vi "Measurement UI.vi"() -> ()   [LabVIEW 2021, in "Sweep_Channel Ganging_UI.lvlib"]
uses:
  Sweep_Channel Ganging_UI.lvlib
panel:
  in  "MeasGraphs":enum32{"I-V Sweep", "Hidden Controls"}(tab)
  out "LoadGraph":T1(graph)
  out "SourceGraph":T2(graph)
  in  "Mode of operation":T3(ring)=enum."Perform measurement"
  out "Source sweep values":dbl[](array[numeric])
  in  "Load measure trigger":string
  in  "Load source trigger":string
  out "Source currents":dbl[](array[numeric])
  out "Source voltages":dbl[](array[numeric])
  out "Load currents":dbl[](array[numeric])
  out "Load voltages":dbl[](array[numeric])
  in  "Load resource names":string[](array[string])
  in  "Source resource names":string[](array[string])
  out "Load sweep points":i32
  out "Source sweep points":i32
  in  "ModeOfConfiguration":T4(tab)
  in  "DEVICE POWER":bool=TRUE
  out "Status":string
  in  "Load config power on":string="Load Config"
  in  "POWERON/OFFLOADResourceNames":refnum<k15>[](array[refnum]) caption="RESOURCE NAMES\n(Single/Master & Slave)"
  in  "Source config power on":string="Source Config"
  in  "POWERON/ OFFSOURCEResourceNames":refnum<k15>[](array[refnum]) caption="RESOURCE NAMES\n(Single/Master & Slave)"
  in  "Power on source sense":i32(ring)=1009 caption="SENSE" items=["Local"=1008, "Remote"=1009]
  in  "Power on/off Source voltage/current limit range":dbl=20.0 caption="CURRENT LIMIT" format="%#_6pA"
  in  "Power on/off Source voltage/current level":dbl=6.0 caption="VOLTAGE LEVEL" format="%#_6pV"
  in  "Power on source system configuration":enum32{"Series", "Parallel"}(ring)=enum."Parallel" caption="SYSTEM CONFIG"
  in  "Power on output function":i32(ring)=1006 caption="OUTPUT FUNCTION" items=["DC Voltage"=1006, "DC Current"=1007]
  in  "MeasConfigurations":enum32{"Source Config", "Load Config"}(tab)
  in  "Measurement timeout":dbl=10.0 caption="MEASUREMENT TIMEOUT" format="%.3ps"
  in  "Source voltage/current compensation frequency":dbl(slide)=3530.0 caption="COMP. FREQUENCY" scale=50.0..1000000.0 scale format="%#_6pHz"
  in  "Source voltage/current pole-zero ratio":dbl(slide)=2.0 caption="POLE-ZERO RATIO" scale=0.0625..16.0
  in  "Source voltage/current gain bandwidth":dbl(slide)=2000.0 caption="GAIN BANDWIDTH" scale=10.0..1000000.0 scale format="%#_6pHz"
  in  "Source enable/disable":bool=TRUE caption="Source Enabled/Disabled"
  in  "Source source delay":dbl=0.005 caption="SOURCE DELAY" format="%.3ps"
  in  "PPSResourceNames":refnum<k15>[](array[refnum]) caption="RESOURCE NAMES\n(Single/Master & Slave)"
  in  "Source stop level":dbl=20.0 caption="STOP LEVEL" format="%#_6pV"
  in  "Source transient response":i32(ring)=1038 caption="TRANSIENT RESPONSE" items=["Slow"=1041, "Normal"=1038, "Fast"=1039, "Custom"=1042]
  in  "Power ON/Source sense":i32(ring)=1009 caption="SENSE" items=["Local"=1008, "Remote"=1009]
  in  "Source voltage/current level range":dbl=20.0 caption="VOLTAGE LEVEL RANGE" format="%#_6pV"
  in  "Power ON V/I Source start level":dbl=6.0 caption="START LEVEL" format="%#_6pV"
  in  "Source current/voltage limit high":dbl=25.0 caption="CURRENT LIMIT/LIMIT HIGH" format="%#_6pA"
  in  "Power ON/Source current/voltage limit range":dbl=25.0 caption="CURRENT LIMIT" format="%#_6pA"
  in  "Source limit symmetry":enum32{"Symmetric", "Asymmetric"}(ring)=enum."Asymmetric" caption="LIMIT SYMMETRY"
  in  "Source current/voltage limit low":dbl=-0.6 caption="CURRENT LIMIT LOW" format="%#_6pA"
  in  "Power ON/Source system configuration":enum32{"Series", "Parallel"}(ring)=enum."Parallel" caption="SYSTEM CONFIG"
  in  "Source compliance":string="Compliance"
  in  "Source sourceadapt":string="SourceAdapt"
  in  "Source sweep points/points per decade":i32=4 caption="PTS/PTS PER DECADE"
  in  "Power ON/Source output function":i32(ring)=1006 caption="OUTPUT FUNCTION" items=["DC Voltage"=1006, "DC Current"=1007]
  in  "Source timing":string="Timings"
  in  "Source aperture time":dbl=0.01666 caption="APERTURE TIME" format="%.3ps"
  in  "Source sweep scale":string(combo)="Linear" caption="SCALE"
  in  "Load Voltage/current compensation frequency":dbl(slide)=250000.0 caption="COMP. FREQUENCY" scale=50.0..1000000.0 scale format="%#_6pHz"
  in  "Load Voltage/current pole-zero ratio":dbl(slide)=5.0 caption="POLE-ZERO RATIO" scale=0.0625..16.0
  in  "Load Voltage/current gain bandwidth":dbl(slide)=50000.0 caption="GAIN BANDWIDTH" scale=10.0..1000000.0 scale format="%#_6pHz"
  in  "Load device voltage/current rating":dbl=30.0 caption="DEVICE CURRENT RATING" format="%#_6pA"
  in  "Load Source Trigger":tag caption="SOURCE TRIGGER"
  in  "Load aperture time":dbl=0.01666 caption="APERTURE TIME" format="%.3ps"
  in  "Load Measure Trigger":tag caption="MEASURE TRIGGER"
  in  "Load trigger config":string="Trigger"
  in  "Load timing":string="Timings"
  in  "Load output function":i32(ring)=1007 caption="OUTPUT FUNCTION" items=["DC Voltage"=1006, "DC Current"=1007]
  in  "Load sweep points/points per decade":i32=10 caption="PTS/PTS PER DECADE"
  in  "Load stop level":dbl=10.0 caption="STOP LEVEL" format="%#_6pA"
  in  "Load sourceadapt":string="SourceAdapt"
  in  "Load compliance":string="Compliance"
  in  "Load system configuration":enum32{"Series", "Parallel"}(ring)=enum."Parallel" caption="SYSTEM CONFIG"
  in  "Load current/voltage limit low":dbl caption="VOLTAGE  LIMIT LOW" format="%#_6pV"
  in  "Load limit symmetry":enum32{"Symmetric", "Asymmetric"}(ring) caption="LIMIT SYMMETRY"
  in  "Load current/voltage limit range":dbl=6.0 caption="VOLTAGE LIMIT RANGE" format="%#_6pV"
  in  "Load current/voltage limit high":dbl=inf caption="VOLTAGE LIMIT/LIMIT HIGH" format="%#_6p"
  in  "Load start level":dbl=2.0 caption="START LEVEL" format="%#_6pA"
  in  "Load voltage/current level range":dbl=80.0 caption="CURRENT LEVEL RANGE" format="%#_6pA"
  in  "Load sense":i32(ring)=1009 caption="SENSE" items=["Local"=1008, "Remote"=1009]
  in  "Load transient response":i32(ring)=1038 caption="TRANSIENT RESPONSE" items=["Slow"=1041, "Normal"=1038, "Fast"=1039, "Custom"=1042]
  in  "LoadResourceNames":refnum<k15>[](array[refnum]) caption="RESOURCE NAMES\n(Single/Master & Slave)"
  in  "Load source delay":dbl=0.005 caption="SOURCE DELAY" format="%.3ps"
  in  "Load sweep scale":string(combo)="Linear" caption="SCALE"
  in  "Load enable/disable":bool=TRUE caption="Load Enabled/Disabled"
  out "Eload status":string
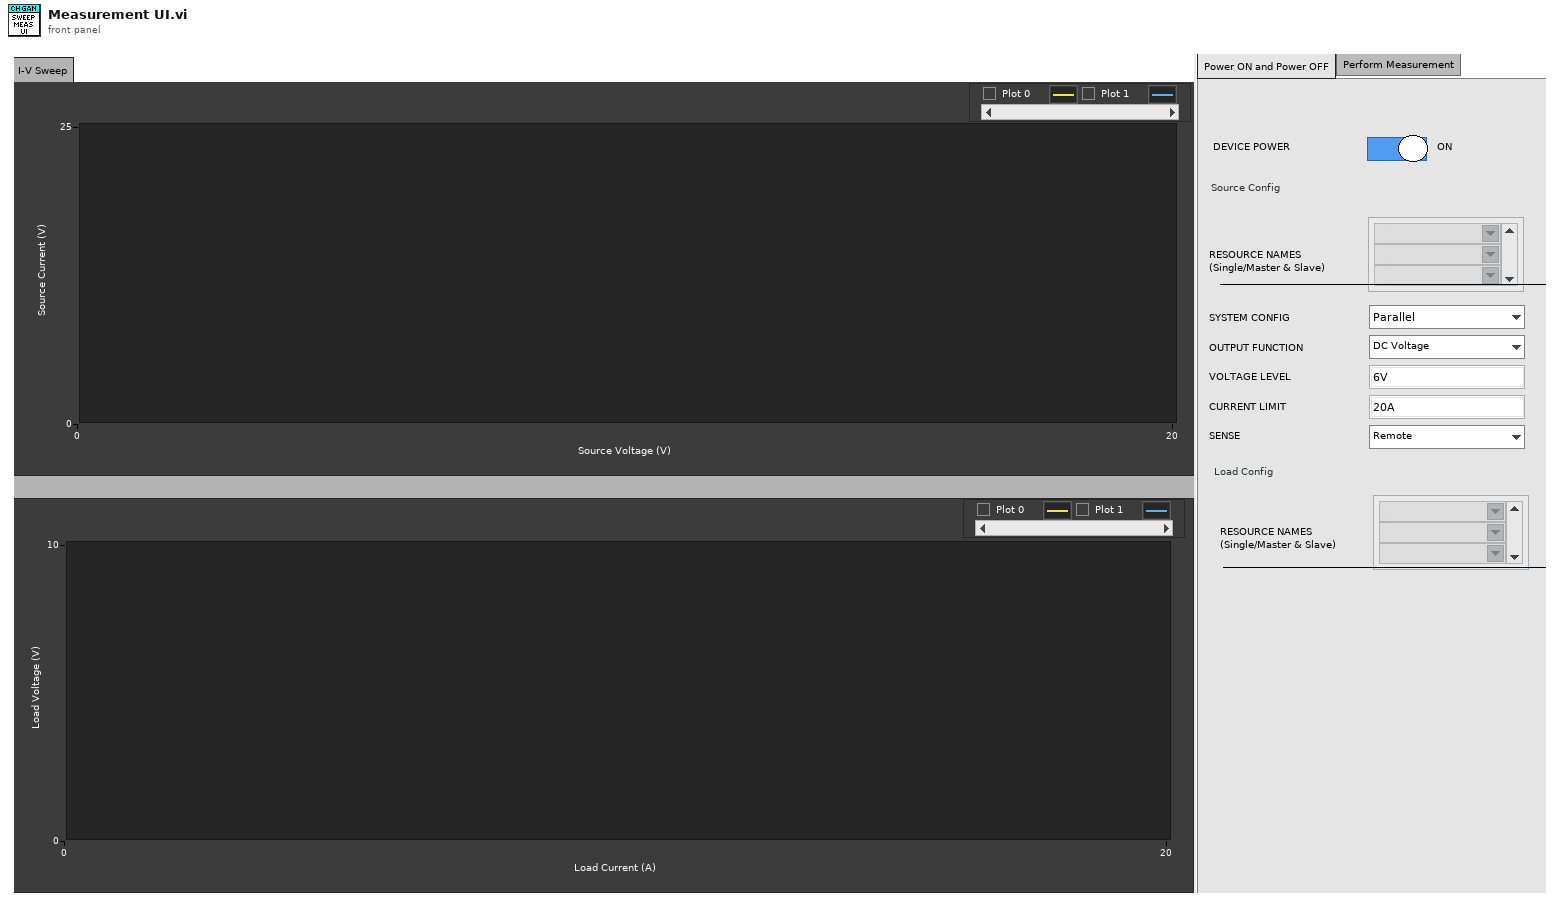
[diagram p1: front panel]
types:
  T1 = cluster{"Ganged load voltages":dbl[], "Ganged load currents":dbl[]}[]
  T2 = cluster{"Ganged source currents":dbl[], "Ganged source voltages":dbl[]}[]
  T3 = enum32{"Power on the DUT", "Perform measurement", "Power off the DUT"}
  T4 = enum32{"Power ON and Power OFF", "Perform Measurement"}
  T5 = enum8{"Enabled", "Disabled", "Disabled and Grayed Out"}
  T6 = cluster{"Source currents":dbl[], "Source voltages":dbl[]}
  T7 = cluster{"Load voltages":dbl[], "Load currents":dbl[]}
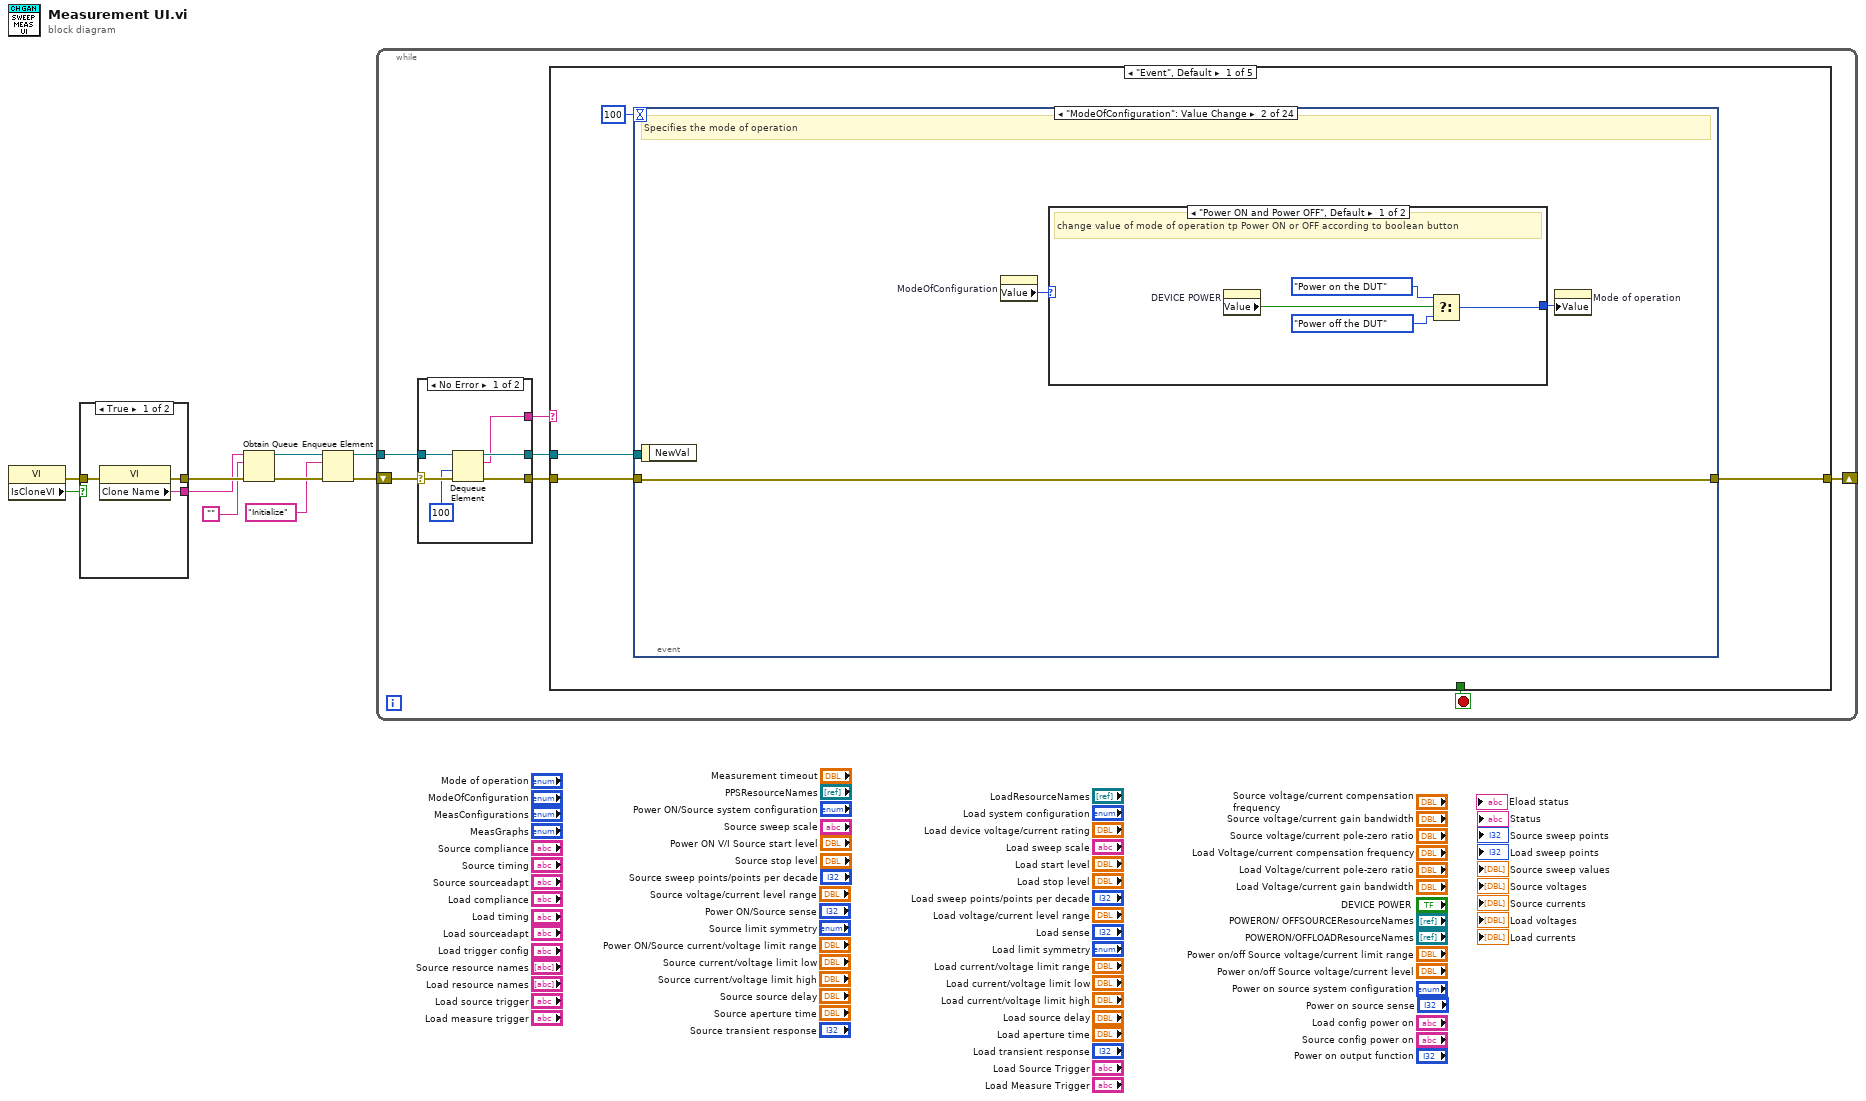
[diagram p0: block diagram]
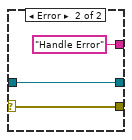
[diagram p2: hidden frame]
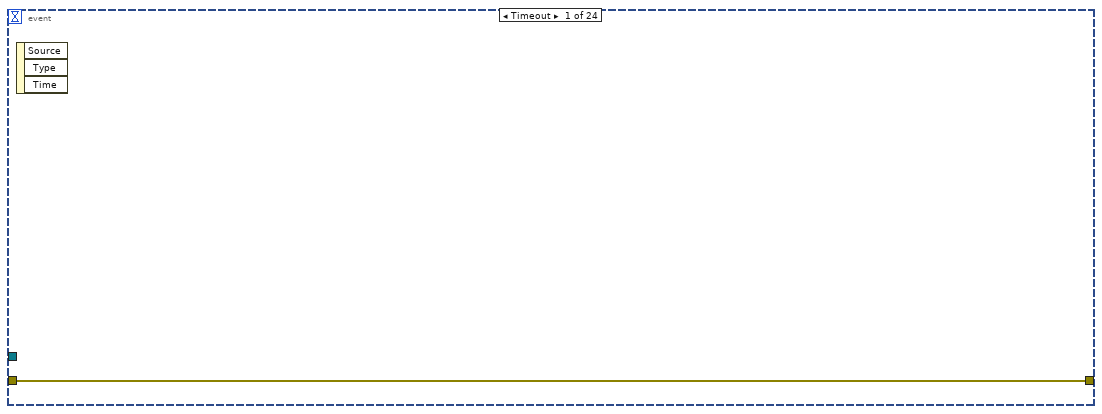
[diagram p3: hidden frame]
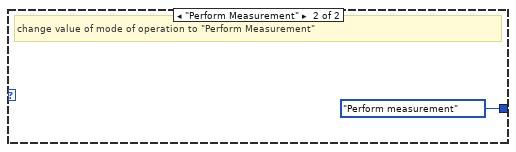
[diagram p4: hidden frame]
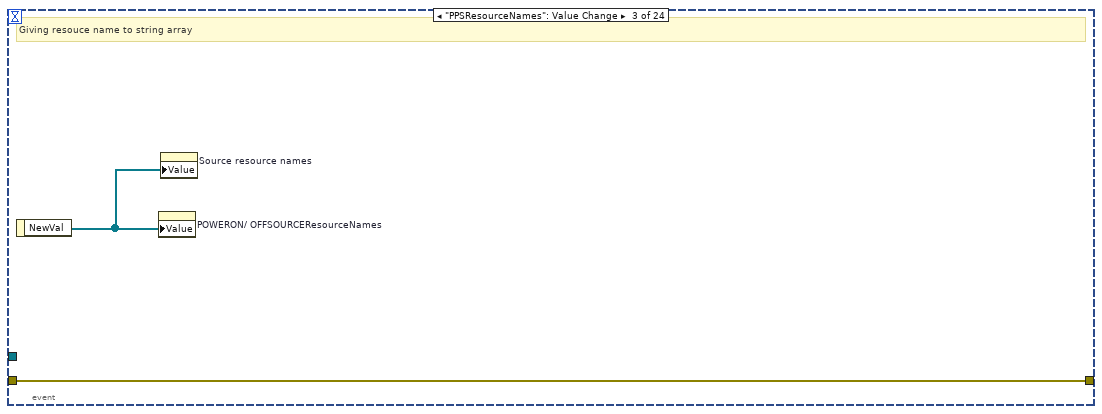
[diagram p5: hidden frame]
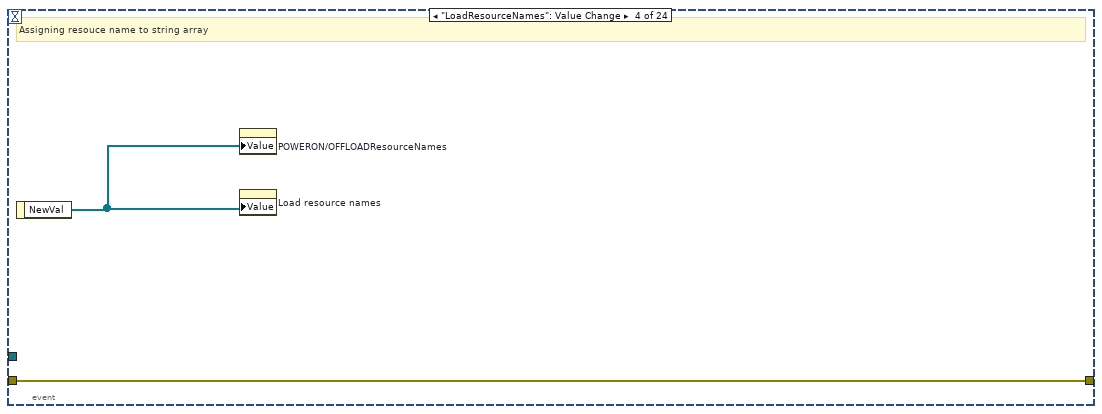
[diagram p6: hidden frame]
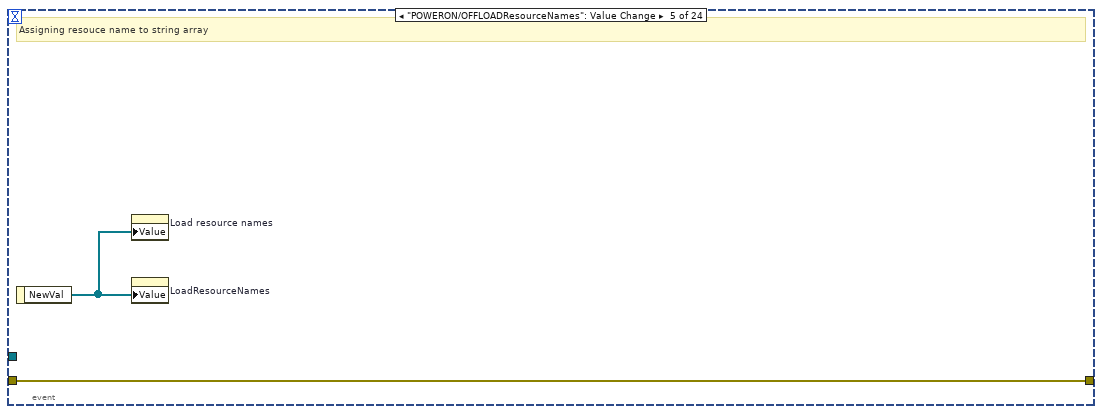
[diagram p7: hidden frame]
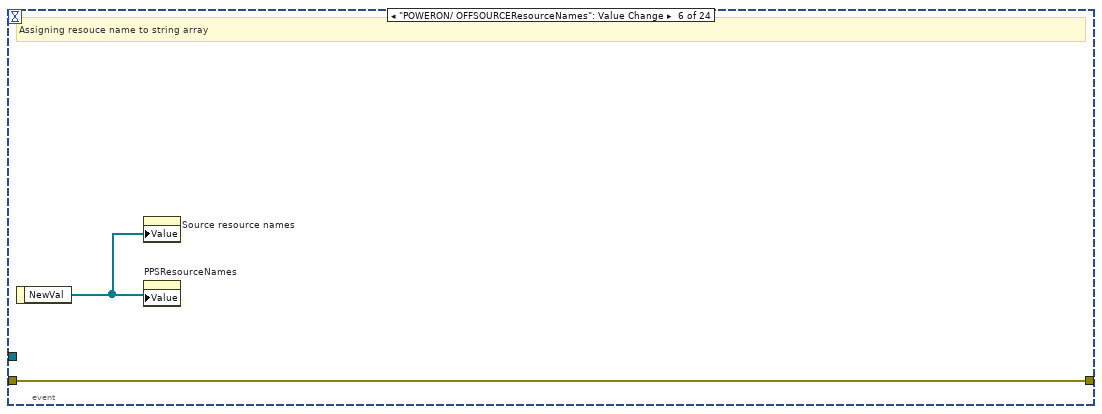
[diagram p8: hidden frame]
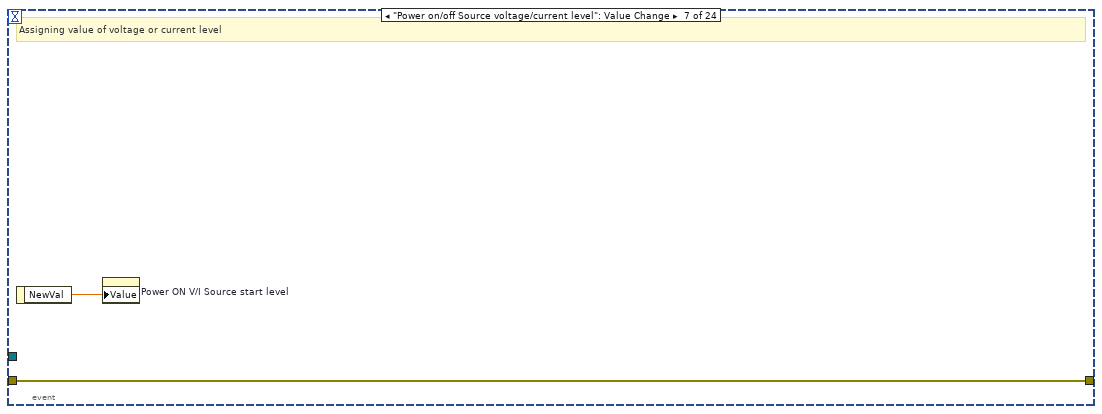
[diagram p9: hidden frame]
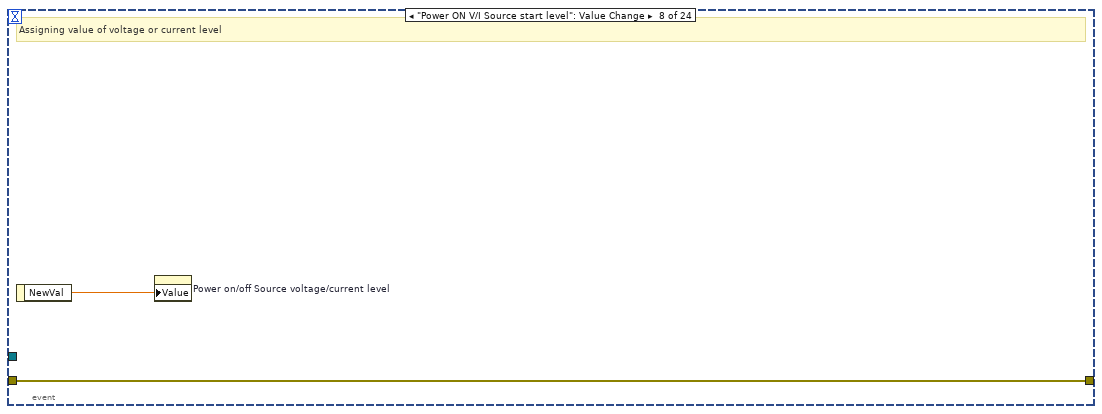
[diagram p10: hidden frame]
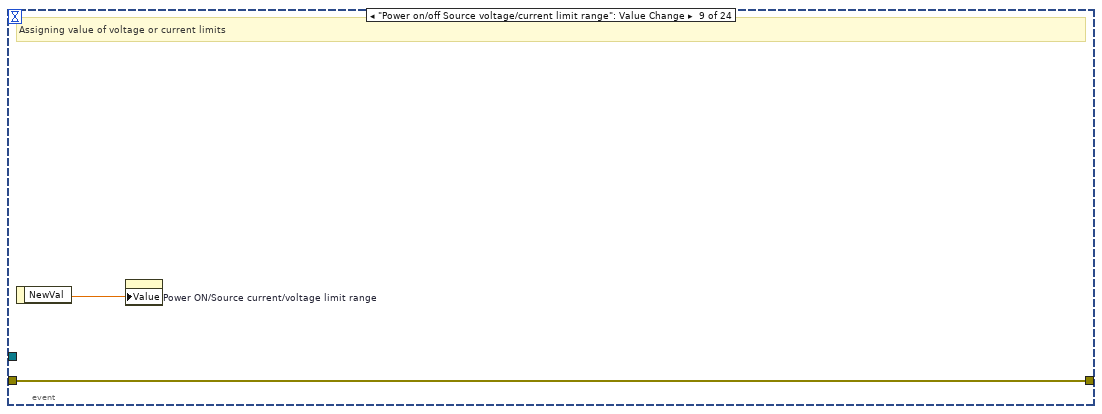
[diagram p11: hidden frame]
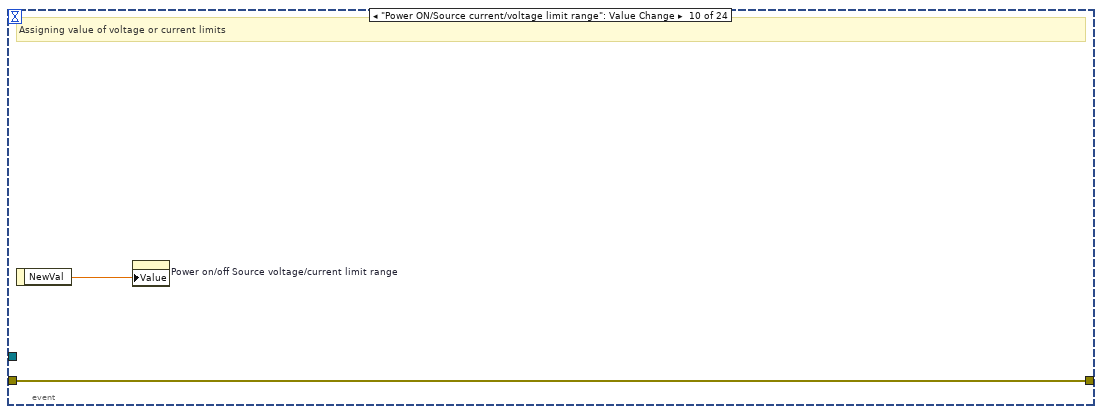
[diagram p12: hidden frame]
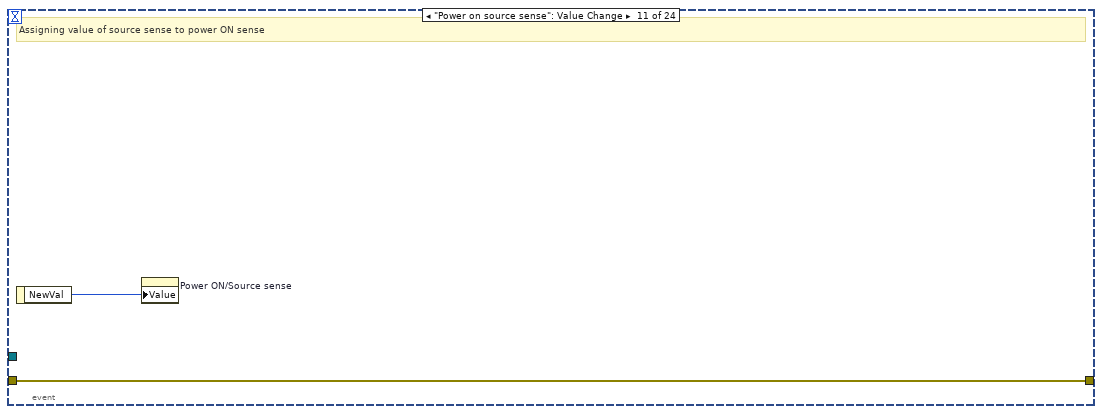
[diagram p13: hidden frame]
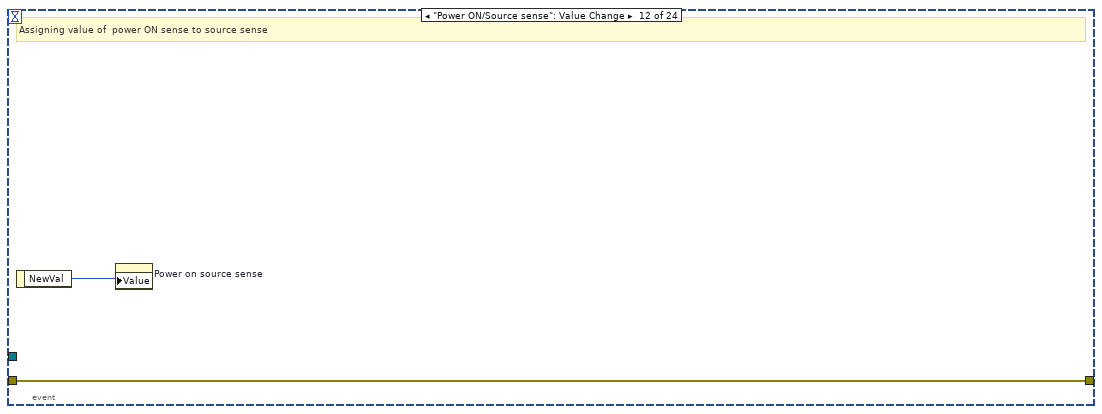
[diagram p14: hidden frame]
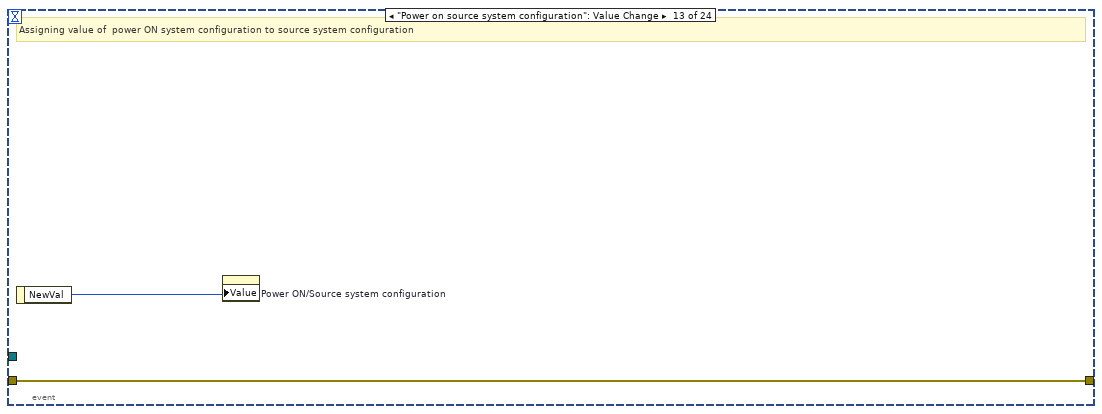
[diagram p15: hidden frame]
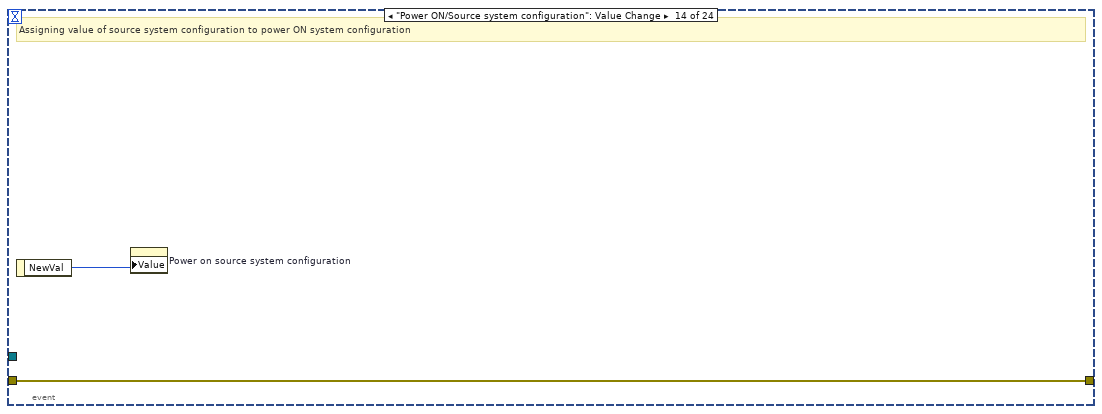
[diagram p16: hidden frame]
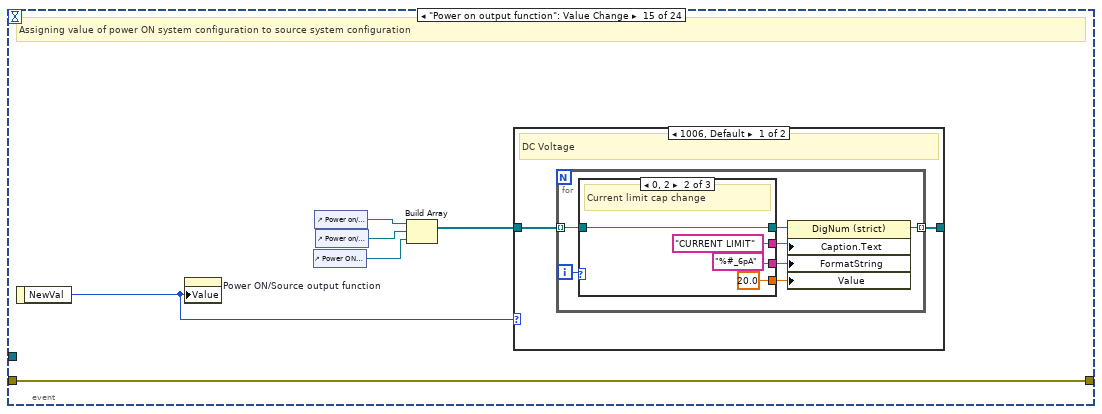
[diagram p17: hidden frame]
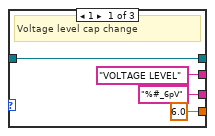
[diagram p18: hidden frame]
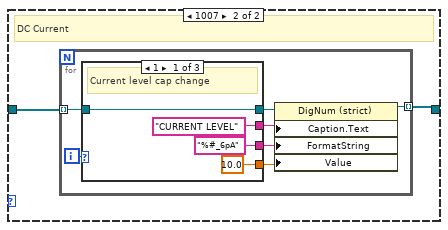
[diagram p20: hidden frame]
diagram:
  n1 = property class="VI"() -> (error out=w1:errorcluster, "IsCloneVI"=w2:bool)  [unwired: 2 in, 1 out]
  n2 = case shown="True" w2 {
    tunnel: [w13 w16] -> w10
    tunnel: [w12 w15] -> w9
    tunnel: w1 -> [w11 w14]
    frame True {
      n3 = property class="VI"(error in=w11) -> (error out=w13:errorcluster, "Clone Name"=w12:string)  [unwired: 1 in, 1 out]
    }
    frame False {
      n4 = property class="VI"(error in=w14) -> (error out=w16:errorcluster, "Name"=w15:string)  [unwired: 1 in, 1 out]
    }
  }
  n5 = Obtain Queue(name (unnamed)=w9, element data type="", error in (no error)=w10) -> (queue out=w6:refnum<queue>, error out=w8:errorcluster)  [unwired: 2 in, 1 out]
  n6 = Enqueue Element(queue=w6, element="Initialize", error in (no error)=w8) -> (queue out=w5:refnum<queue>, error out=w7:errorcluster)  [unwired: 1 in, 1 out]
  n7 = while {
    shift-right: [w18] -> _
    shift-left: w7 -> [w23]
    tunnel: w5 -> [w21]
    stop <- w17 stop-if-true
    n8 = case shown="No Error" w23 {
      selector: w23 -> [w29 w32]
      tunnel: [w28 w32] -> w22
      tunnel: w21 -> [w27 w31]
      tunnel: [w26 w31] -> w20
      tunnel: [w25 "Handle Error"] -> w19
      frame No Error {
        n9 = Dequeue Element(queue=w27, timeout in ms (-1)=100, error in (no error)=w29) -> (queue out=w26:refnum<queue>, element=w25:string, error out=w28:errorcluster)  [unwired: 1 out]
      }
      frame Error {
      }
    }
    n10 = case shown="\"Event\", Default" w19 {
      tunnel: w22 -> [w35 w303 w333 w401 w402]
      tunnel: w20 -> [w33 _ _ w399 _]
      tunnel: [w36 w303 w333 w396 w402] -> w18
      tunnel: [_ _ _ TRUE _] -> w17
      frame "Event", Default {
        n11 = event shown="[1] \"ModeOfConfiguration\": Value Change" {
          selector: _ -> [_ _ _ _ _ _ _ _ _ _ _ _ _ _ _ _ _ _ _ _ _ _ _ _]
          dyn-events: _ -> [_ _ _ _ _ _ _ _ _ _ _ _ _ _ _ _ _ _ _ _ _ _ _ _]
          timeout: 100 -> [_ _ _ _ _ _ _ _ _ _ _ _ _ _ _ _ _ _ _ _ _ _ _ _]
          tunnel: [w37 w38 w47 w49 w51 w53 w55 w57 w58 w61 w62 w64 w66 w68 w75 w111 w188 w274 w276 w278 w283 _ _ w298] -> w36
          tunnel: w35 -> [w37 w38 w47 w49 w51 w53 w55 w57 w58 w61 w62 w64 w66 w68 w75 w112 w189 w274 w276 w278 w283 _ _ w299]
          tunnel: w33 -> [_ _ _ _ _ _ _ _ _ _ _ _ _ _ _ _ _ _ _ _ _ _ _ w297]
          event Timeout {
            n12 = event-data() -> ()  [unwired: 1 in, 3 out]
          }
          event "ModeOfConfiguration": Value Change {
            # "Specifies the mode of operation"
            n13 = event-data() -> ()  [unwired: 1 in, 1 out]
            n14 = property on="ModeOfConfiguration" class="TabCtl (strict)"() -> ("Value"=w40:T4)  [unwired: 2 in, 2 out]
            n15 = case shown="\"Power ON and Power OFF\", Default" w40 {
              tunnel: [w43 T3."Perform measurement" ("Mode of operation")] -> w39
              frame "Power ON and Power OFF", Default {
                # "change value of mode of operation tp Power ON or OFF according to boolean button"
                n16 = property on="DEVICE POWER" class="Bool (strict)"() -> ("Value"=w41:bool)  [unwired: 2 in, 2 out]
                n17 = Select(t=T3."Power on the DUT" ("Mode of operation"), s=w41, f=T3."Power off the DUT" ("Mode of operation")) -> (s? t:f=w43:T3)
              }
              frame "Perform Measurement" {
                # "change value of mode of operation to \"Perform Measurement\""
              }
            }
            n18 = property on="Mode of operation" class="Enum (strict)"("Value"=w39) -> ()  [unwired: 2 in, 2 out]
          }
          event "PPSResourceNames": Value Change {
            # "Giving resouce name to string array"
            n19 = event-data() -> ("NewVal"=w46:refnum<k15>[])  [unwired: 1 in]
            n20 = property on="POWERON/ OFFSOURCEResourceNames" class="Arr (strict)"("Value"=w46) -> ()  [unwired: 2 in, 2 out]
            n21 = property on="Source resource names" class="Arr (strict)"("Value"=w46) -> ()  [unwired: 2 in, 2 out]
          }
          event "LoadResourceNames": Value Change {
            # "Assigning resouce name to string array"
            n22 = event-data() -> ("NewVal"=w48:refnum<k15>[])  [unwired: 1 in]
            n23 = property on="POWERON/OFFLOADResourceNames" class="Arr (strict)"("Value"=w48) -> ()  [unwired: 2 in, 2 out]
            n24 = property on="Load resource names" class="Arr (strict)"("Value"=w48) -> ()  [unwired: 2 in, 2 out]
          }
          event "POWERON/OFFLOADResourceNames": Value Change {
            # "Assigning resouce name to string array"
            n25 = event-data() -> ("NewVal"=w50:refnum<k15>[])  [unwired: 1 in]
            n26 = property on="Load resource names" class="Arr (strict)"("Value"=w50) -> ()  [unwired: 2 in, 2 out]
            n27 = property on="LoadResourceNames" class="Arr (strict)"("Value"=w50) -> ()  [unwired: 2 in, 2 out]
          }
          event "POWERON/ OFFSOURCEResourceNames": Value Change {
            # "Assigning resouce name to string array"
            n28 = event-data() -> ("NewVal"=w52:refnum<k15>[])  [unwired: 1 in]
            n29 = property on="Source resource names" class="Arr (strict)"("Value"=w52) -> ()  [unwired: 2 in, 2 out]
            n30 = property on="PPSResourceNames" class="Arr (strict)"("Value"=w52) -> ()  [unwired: 2 in, 2 out]
          }
          event "Power on/off Source voltage/current level": Value Change {
            # "Assigning value of voltage or current level"
            n31 = event-data() -> ("NewVal"=w54:dbl)  [unwired: 1 in]
            n32 = property on="Power ON V/I Source start level" class="DigNum (strict)"("Value"=w54) -> ()  [unwired: 2 in, 2 out]
          }
          event "Power ON V/I Source start level": Value Change {
            # "Assigning value of voltage or current level"
            n33 = event-data() -> ("NewVal"=w56:dbl)  [unwired: 1 in]
            n34 = property on="Power on/off Source voltage/current level" class="DigNum (strict)"("Value"=w56) -> ()  [unwired: 2 in, 2 out]
          }
          event "Power on/off Source voltage/current limit range": Value Change {
            # "Assigning value of voltage or current limits"
            n35 = event-data() -> ("NewVal"=w59:dbl)  [unwired: 1 in]
            n36 = property on="Power ON/Source current/voltage limit range" class="DigNum (strict)"("Value"=w59) -> ()  [unwired: 2 in, 2 out]
          }
          event "Power ON/Source current/voltage limit range": Value Change {
            # "Assigning value of voltage or current limits"
            n37 = event-data() -> ("NewVal"=w60:dbl)  [unwired: 1 in]
            n38 = property on="Power on/off Source voltage/current limit range" class="DigNum (strict)"("Value"=w60) -> ()  [unwired: 2 in, 2 out]
          }
          event "Power on source sense": Value Change {
            # "Assigning value of source sense to power ON sense"
            n39 = event-data() -> ("NewVal"=w63:i32)  [unwired: 1 in]
            n40 = property on="Power ON/Source sense" class="Ring (strict)"("Value"=w63) -> ()  [unwired: 2 in, 2 out]
          }
          event "Power ON/Source sense": Value Change {
            # "Assigning value of  power ON sense to source sense"
            n41 = event-data() -> ("NewVal"=w65:i32)  [unwired: 1 in]
            n42 = property on="Power on source sense" class="Ring (strict)"("Value"=w65) -> ()  [unwired: 2 in, 2 out]
          }
          event "Power on source system configuration": Value Change {
            # "Assigning value of  power ON system configuration to source system configuration"
            n43 = event-data() -> ("NewVal"=w67:enum32{"Series", "Parallel"})  [unwired: 1 in]
            n44 = property on="Power ON/Source system configuration" class="Enum (strict)"("Value"=w67) -> ()  [unwired: 2 in, 2 out]
          }
          event "Power ON/Source system configuration": Value Change {
            # "Assigning value of source system configuration to power ON system configuration"
            n45 = event-data() -> ("NewVal"=w69:enum32{"Series", "Parallel"})  [unwired: 1 in]
            n46 = property on="Power on source system configuration" class="Enum (strict)"("Value"=w69) -> ()  [unwired: 2 in, 2 out]
          }
          event "Power on output function": Value Change {
            # "Assigning value of power ON system configuration to source system configuration"
            n47 = event-data() -> ("NewVal"=w74:i32)  [unwired: 1 in]
            n48 = property on="Power ON/Source output function" class="Ring (strict)"("Value"=w74) -> ()  [unwired: 2 in, 2 out]
            n49 = control-ref of="Power ON/Source current/voltage limit range"() -> (w70:refnum<vi>)
            n50 = control-ref of="Power on/off Source voltage/current limit range"() -> (w73:refnum<vi>)
            n51 = control-ref of="Power on/off Source voltage/current level"() -> (w72:refnum<vi>)
            n52 = Build Array(w73, w72, w70) -> (w71:refnum<vi>[])
            n53 = case shown="1006, Default" w74 {
              tunnel: w71 -> [w77 w94]
              tunnel: [w76 w93] -> _
              frame 1006, Default {
                # "DC Voltage"
                n54 = for {
                  tunnel: w77 -> [w82] mode=indexing
                  tunnel: [w78] -> w76 mode=indexing
                  i -> [w84]
                  n55 = case shown="0, 2" w84 {
                    tunnel: [w88 w92 _] -> w83
                    tunnel: w82 -> [w88 w92 _]
                    tunnel: ["VOLTAGE LEVEL" ("Caption.Text") "CURRENT LIMIT" ("Caption.Text") _] -> w81
                    tunnel: ["%#_6pV" ("Format String") "%#_6pA" ("Format String") _] -> w80
                    tunnel: [6.0 ("Value") 20.0 ("Value") _] -> w79
                    frame 1 {
                      # "Voltage level cap change"
                    }
                    frame 0, 2 {
                      # "Current limit cap change"
                    }
                    frame Default {
                    }
                  }
                  n56 = property class="DigNum (strict)"(reference=w83, "Caption.Text"=w81, "FormatString"=w80, "Value"=w79) -> (reference out=w78:refnum<vi>)  [unwired: 1 in, 1 out]
                }
              }
              frame 1007 {
                # "DC Current"
                n57 = for {
                  tunnel: w94 -> [w99] mode=indexing
                  tunnel: [w95] -> w93 mode=indexing
                  i -> [w101]
                  n58 = case shown="1" w101 {
                    tunnel: [w105 w109 _] -> w100
                    tunnel: w99 -> [w105 w109 _]
                    tunnel: ["CURRENT LEVEL" ("Caption.Text") "VOLTAGE LIMIT" ("Caption.Text") _] -> w98
                    tunnel: ["%#_6pA" ("Format String") "%#_6pV" ("Format String") _] -> w97
                    tunnel: [10.0 ("Value") 20.0 ("Value") _] -> w96
                    frame 1 {
                      # "Current level cap change"
                    }
                    frame 0, 2 {
                      # "Voltage limit cap change"
                    }
                    frame Default {
                    }
                  }
                  n59 = property class="DigNum (strict)"(reference=w100, "Caption.Text"=w98, "FormatString"=w97, "Value"=w96) -> (reference out=w95:refnum<vi>)  [unwired: 1 in, 1 out]
                }
              }
            }
          }
          event "Power ON/Source output function": Value Change {
            # "Assigning value of source system configuration to power ON system configuration and change in caption of few of the controls"
            n60 = event-data() -> ("NewVal"=w110:i32)  [unwired: 1 in]
            n61 = property on="Power on output function" class="Ring (strict)"("Value"=w110) -> ()  [unwired: 2 in, 2 out]
            n62 = control-ref of="Power ON V/I Source start level"() -> (w120:refnum<vi>)
            n63 = control-ref of="Source stop level"() -> (w119:refnum<vi>)
            n64 = control-ref of="Source voltage/current level range"() -> (w118:refnum<vi>)
            n65 = control-ref of="Power ON/Source current/voltage limit range"() -> (w117:refnum<vi>)
            n66 = control-ref of="Source current/voltage limit low"() -> (w116:refnum<vi>)
            n67 = control-ref of="Source current/voltage limit high"() -> (w115:refnum<vi>)
            n68 = Build Array(w120, w119, w118, w117, w116, w115) -> (w114:refnum<vi>[])
            n69 = case shown="1006, Default" w110 {
              tunnel: w114 -> [w122 w155]
              tunnel: [w121 w154] -> w113
              frame 1006, Default {
                # "DC Voltage"
                n70 = for {
                  tunnel: w122 -> [w127] mode=indexing
                  tunnel: [w123] -> w121 mode=indexing
                  i -> [w129]
                  n71 = case shown="3" w129 {
                    tunnel: [w133 w137 w141 w145 w148 w152 _] -> w128
                    tunnel: w127 -> [w133 w137 w141 w145 w148 w152 _]
                    tunnel: ["START LEVEL" ("Caption.Text") "STOP LEVEL" ("Caption.Text") "VOLTAGE LEVEL RANGE" ("Caption.Text") "CURRENT LIMIT RANGE" ("Caption.Text") "CURRENT LIMIT LOW" ("Caption.Text") "CURRENT LIMIT/LIMIT HIGH" ("Caption.Text") _] -> w126
                    tunnel: ["%#_6pV" ("Format String") "%#_6pV" ("Format String") "%#_6pV" ("Format String") "%#_6pA" ("Format String") "%#_6pA" ("Format String") "%#_6pA" ("Format String") _] -> w125
                    tunnel: [1.0 ("Value") 20.0 ("Value") 20.0 ("Value") 15.0 ("Value") -0.6 ("Value") 15.0 ("Value") _] -> w124
                    frame 0 {
                      # "Start voltage level cap change"
                    }
                    frame 1 {
                      # "Stop voltage level cap change"
                    }
                    frame 2 {
                      # "Voltage level range cap change"
                    }
                    frame 3 {
                      # "Current limit range cap change"
                    }
                    frame 4 {
                      # "Current limit low cap change"
                    }
                    frame 5 {
                      # "Current limit high cap change"
                    }
                    frame Default {
                    }
                  }
                  n72 = property class="DigNum (strict)"(reference=w128, "Caption.Text"=w126, "FormatString"=w125, "Value"=w124) -> (reference out=w123:refnum<vi>)  [unwired: 1 in, 1 out]
                }
              }
              frame 1007 {
                # "DC Current"
                n73 = for {
                  tunnel: w155 -> [w160] mode=indexing
                  tunnel: [w156] -> w154 mode=indexing
                  i -> [w162]
                  n74 = case shown="3" w162 {
                    tunnel: [w166 w170 w174 w178 w181 w185 _] -> w161
                    tunnel: w160 -> [w166 w170 w174 w178 w181 w185 _]
                    tunnel: ["START LEVEL" ("Caption.Text") "STOP LEVEL" ("Caption.Text") "CURRENT LEVEL RANGE" ("Caption.Text") "VOLTAGE LIMIT RANGE" ("Caption.Text") "VOLTAGE  LIMIT LOW" ("Caption.Text") "VOLTAGE LIMIT/LIMIT HIGH" ("Caption.Text") _] -> w159
                    tunnel: ["%#_6pA" ("Format String") "%#_6pA" ("Format String") "%#_6pA" ("Format String") "%#_6pV" ("Format String") "%#_6pV" ("Format String") "%#_6pV" ("Format String") _] -> w158
                    tunnel: [1.0 ("Value") 25.0 ("Value") 25.0 ("Value") 12.0 ("Value") -0.6 ("Value") 12.0 ("Value") _] -> w157
                    frame 0 {
                      # "Current start level cap change"
                    }
                    frame 1 {
                      # "Current stop level cap change"
                    }
                    frame 2 {
                      # "Current level range cap change"
                    }
                    frame 3 {
                      # "Voltage limit range cap change"
                    }
                    frame 4 {
                      # "Voltage limit low cap change"
                    }
                    frame 5 {
                      # "Voltage limit high cap change"
                    }
                    frame Default {
                    }
                  }
                  n75 = property class="DigNum (strict)"(reference=w161, "Caption.Text"=w159, "FormatString"=w158, "Value"=w157) -> (reference out=w156:refnum<vi>)  [unwired: 1 in, 1 out]
                }
              }
            }
            n76 = Close Reference(reference=w113, error in (no error)=w112) -> (error out=w111:errorcluster)
          }
          event "Load output function": Value Change {
            # "Change in caption of few of the controls"
            n77 = event-data() -> ("NewVal"=w198:i32)  [unwired: 1 in]
            n78 = control-ref of="Load device voltage/current rating"() -> (w187:refnum<vi>)
            n79 = control-ref of="Load start level"() -> (w197:refnum<vi>)
            n80 = control-ref of="Load stop level"() -> (w196:refnum<vi>)
            n81 = control-ref of="Load voltage/current level range"() -> (w194:refnum<vi>)
            n82 = control-ref of="Load current/voltage limit range"() -> (w193:refnum<vi>)
            n83 = control-ref of="Load current/voltage limit low"() -> (w192:refnum<vi>)
            n84 = control-ref of="Load current/voltage limit high"() -> (w191:refnum<vi>)
            n85 = Build Array(w197, w196, w194, w193, w192, w191, w187) -> (w195:refnum<vi>[])
            n86 = case shown="1007, Default" w198 {
              tunnel: w195 -> [w200 w237]
              tunnel: [w199 w236] -> w190
              frame 1006 {
                # "DC Voltage"
                n87 = for {
                  tunnel: w200 -> [w205] mode=indexing
                  tunnel: [w201] -> w199 mode=indexing
                  i -> [w207]
                  n88 = case shown="0" w207 {
                    tunnel: [w211 w215 w219 w223 w226 w230 w235 _] -> w206
                    tunnel: w205 -> [w211 w215 w219 w223 w226 w230 w235 _]
                    tunnel: ["START LEVEL" ("Caption.Text") "STOP LEVEL" ("Caption.Text") "VOLTAGE LEVEL RANGE" ("Caption.Text") "CURRENT LIMIT RANGE" ("Caption.Text") "CURRENT LIMIT LOW" ("Caption.Text") "CURRENT LIMIT/LIMIT HIGH" ("Caption.Text") "DEVICE VOLTAGE RATING" ("Caption.Text") _] -> w204
                    tunnel: ["%#_6pV" ("Format String") "%#_6pV" ("Format String") "%#_6pV" ("Format String") "%#_6pA" ("Format String") "%#_6pA" ("Format String") "%#_6pA" ("Format String") "%#_6pV" ("Format String") _] -> w203
                    tunnel: [1.0 ("Value") 60.0 ("Value") 60.0 ("Value") 4.0 ("Value") 0.0 ("Value") 4.0 ("Value") 25.0 ("Value") _] -> w202
                    frame 0 {
                      # "Start voltage level cap change"
                    }
                    frame 1 {
                      # "Stop voltage level cap change"
                    }
                    frame 2 {
                      # "Voltage level range cap change"
                    }
                    frame 3 {
                      # "Current limit range cap change"
                    }
                    frame 4 {
                      # "Current limit low cap change"
                    }
                    frame 5 {
                      # "Current limit high cap change"
                    }
                    frame 6 {
                      # "Device rating cap change"
                    }
                    frame Default {
                    }
                  }
                  n89 = property class="DigNum (strict)"(reference=w206, "Caption.Text"=w204, "FormatString"=w203, "Value"=w202) -> (reference out=w201:refnum<vi>)  [unwired: 1 in, 1 out]
                }
              }
              frame 1007, Default {
                # "DC Current"
                n90 = for {
                  tunnel: w237 -> [w242] mode=indexing
                  tunnel: [w238] -> w236 mode=indexing
                  i -> [w244]
                  n91 = case shown="0" w244 {
                    tunnel: [w248 w252 w256 w260 w263 w268 w271 _] -> w243
                    tunnel: w242 -> [w248 w252 w256 w260 w263 w268 w271 _]
                    tunnel: ["START LEVEL" ("Caption.Text") "STOP LEVEL" ("Caption.Text") "CURRENT LEVEL RANGE" ("Caption.Text") "VOLTAGE LIMIT RANGE" ("Caption.Text") "VOLTAGE  LIMIT LOW" ("Caption.Text") "VOLTAGE LIMIT/LIMIT HIGH" ("Caption.Text") "DEVICE CURRENT RATING" ("Caption.Text") _] -> w241
                    tunnel: ["%#_6pA" ("Format String") "%#_6pA" ("Format String") "%#_6pA" ("Format String") "%#_6pV" ("Format String") "%#_6pV" ("Format String") "%#_6p" ("Format String") "%#_6pA" ("Format String") _] -> w240
                    tunnel: [1.0 ("Value") 40.0 ("Value") 40.0 ("Value") 6.0 ("Value") 0.0 ("Value") w266 30.0 ("Value") _] -> w239
                    frame 0 {
                      # "Start current level cap change"
                    }
                    frame 1 {
                      # "Stop current level cap change"
                    }
                    frame 2 {
                      # "Current level range cap change"
                    }
                    frame 3 {
                      # "Voltage limit range cap change"
                    }
                    frame 4 {
                      # "Voltage limit low cap change"
                    }
                    frame 5 {
                      # "Voltage limit high cap change"
                      n92 = Reciprocal(x=0.0) -> (1/x=w266:dbl)
                    }
                    frame 6 {
                      # "Device rating cap change"
                    }
                    frame Default {
                    }
                  }
                  n93 = property class="DigNum (strict)"(reference=w243, "Caption.Text"=w241, "FormatString"=w240, "Value"=w239) -> (reference out=w238:refnum<vi>)  [unwired: 1 in, 1 out]
                }
              }
            }
            n94 = Close Reference(reference=w190, error in (no error)=w189) -> (error out=w188:errorcluster)
          }
          event "Load Source Trigger": Value Change {
            # "Giving value of load trigger to string load source trigger"
            n95 = event-data() -> ("NewVal"=w275:tag)  [unwired: 1 in]
            n96 = property on="Load source trigger" class="Str"("Value"=w275) -> ()  [unwired: 2 in, 2 out]
          }
          event "Load Measure Trigger": Value Change {
            # "Giving value of load trigger to string load measure trigger"
            n97 = event-data() -> ("NewVal"=w277:tag)  [unwired: 1 in]
            n98 = property on="Load measure trigger" class="Str"("Value"=w277) -> ()  [unwired: 2 in, 2 out]
          }
          event "Source sweep scale": Value Change {
            # "changing the scale of source X-Scale according to the sweep type"
            n99 = event-data() -> ("NewVal"=w280:string)  [unwired: 1 in]
            n100 = case shown="\"Logarithmic\"" w280 {
              tunnel: [u8 0 ("X Scale.Mapping Mode") u8 1 ("X Scale.Mapping Mode")] -> w279
              frame "Linear", Default {
              }
              frame "Logarithmic" {
              }
            }
            n101 = property on="SourceGraph" class="XYGraph (strict)"("XScale.Mapping Mode"=w279) -> ()  [unwired: 2 in, 2 out]
          }
          event "Load sweep scale": Value Change {
            # "changing the scale of load X-Scale according to the sweep type"
            n102 = event-data() -> ("NewVal"=w285:string)  [unwired: 1 in]
            n103 = case shown="\"Logarithmic\"" w285 {
              tunnel: [u8 0 ("X Scale.Mapping Mode") u8 1 ("X Scale.Mapping Mode")] -> w284
              frame "Linear", Default {
              }
              frame "Logarithmic" {
              }
            }
            n104 = property on="LoadGraph" class="XYGraph (strict)"("XScale.Mapping Mode"=w284) -> ()  [unwired: 2 in, 2 out]
          }
          event "Load transient response": Value Change {
            # "Disabling and enabling transient parameter according to transient response control value"
            n105 = event-data() -> ("NewVal"=w289:i32)  [unwired: 1 in]
            n106 = case shown="1042" w289 {
              tunnel: [T5."Disabled and Grayed Out" ("Disabled") T5."Enabled" ("Disabled")] -> w288
              frame 1038, 1039, 1041, Default {
                # "Slow, Normal and Fast transient disables and grey out the following controls"
              }
              frame 1042 {
                # "Custom transient enables the following controls"
              }
            }
            n107 = property on="Load Voltage/current compensation frequency" class="Slide (strict)"("DisabledEnum"=w288) -> ()  [unwired: 2 in, 2 out]
            n108 = property on="Load Voltage/current pole-zero ratio" class="Slide (strict)"("DisabledEnum"=w288) -> ()  [unwired: 2 in, 2 out]
            n109 = property on="Load Voltage/current gain bandwidth" class="Slide (strict)"("DisabledEnum"=w288) -> ()  [unwired: 2 in, 2 out]
          }
          event "Source transient response": Value Change {
            # "Disabling and enabling transient parameter according to transient response control value"
            n110 = event-data() -> ("NewVal"=w293:i32)  [unwired: 1 in]
            n111 = case shown="1042" w293 {
              tunnel: [T5."Disabled and Grayed Out" ("Disabled") T5."Enabled" ("Disabled")] -> w292
              frame 1038, 1039, 1041, Default {
                # "Slow, Normal and Fast transient disables and grey out the following controls"
              }
              frame 1042 {
                # "Custom transient enables the following controls"
              }
            }
            n112 = property on="Source voltage/current compensation frequency" class="Slide (strict)"("DisabledEnum"=w292) -> ()  [unwired: 2 in, 2 out]
            n113 = property on="Source voltage/current gain bandwidth" class="Slide (strict)"("DisabledEnum"=w292) -> ()  [unwired: 2 in, 2 out]
            n114 = property on="Source voltage/current pole-zero ratio" class="Slide (strict)"("DisabledEnum"=w292) -> ()  [unwired: 2 in, 2 out]
          }
          event Panel Close? {
            n115 = event-data() -> ()  [unwired: 1 in, 4 out]
            n116 = Enqueue Element(queue=w297, element="Exit", error in (no error)=w299) -> (error out=w298:errorcluster)  [unwired: 1 in, 2 out]
            n117 = event-data("Discard?"=TRUE) -> ()  [unwired: 1 in, 1 out]
          }
        }
      }
      frame "Initialize" {
        n118 = property on="ModeOfConfiguration" class="TabCtl (strict)"("Value"=T4."Power ON and Power OFF" ("ModeOfConfiguration")) -> ()  [unwired: 2 in, 2 out]
        n119 = property on="Status" class="Str"("Value"="" ("Status")) -> ()  [unwired: 2 in, 2 out]
      }
      frame "Post UI Update" {
        # "Change the X-Scale and Y-Scale label according to the output function given."
        # "This case will be triggered, after framework updates the User interface with result values."
        n120 = local read "Source voltages"() -> (w329:dbl[])
        n121 = local read "Source currents"() -> (w327:dbl[])
        n122 = local read "Load currents"() -> (w324:dbl[])
        n123 = local read "Load voltages"() -> (w323:dbl[])
        n124 = case shown="1006, Default" "Power ON/Source output function" {
          tunnel: w329 -> [w374 w378]
          tunnel: [w374 w377] -> w328
          tunnel: w327 -> [w373 w377]
          tunnel: [w373 w378] -> w326
          tunnel: ["Source Voltage (V)" ("X Scale.Name Label.Text") "Source Current (A)" ("X Scale.Name Label.Text")] -> w321
          tunnel: ["Source Current (A)" ("X Scale.Name Label.Text") "Source Voltage (V)" ("X Scale.Name Label.Text")] -> w320
          frame 1006, Default {
          }
          frame 1007 {
          }
        }
        n125 = case shown="1007, Default" "Load output function" {
          tunnel: w324 -> [w366 w368]
          tunnel: [w366 w367] -> w325
          tunnel: w323 -> [w365 w367]
          tunnel: [w365 w368] -> w322
          tunnel: ["Load Current (A)" ("X Scale.Name Label.Text") "Load Voltage (V)" ("X Scale.Name Label.Text")] -> w319
          tunnel: ["Load Voltage (V)" ("X Scale.Name Label.Text") "Load Current (A)" ("X Scale.Name Label.Text")] -> w318
          frame 1007, Default {
          }
          frame 1006 {
          }
        }
        n126 = property on="LoadGraph" class="XYGraph (strict)"("XScale.NameLbl.Text"=w319, "YScale.NameLbl.Text"=w318) -> ()  [unwired: 2 in, 2 out]
        n127 = property on="SourceGraph" class="XYGraph (strict)"("XScale.NameLbl.Text"=w321, "YScale.NameLbl.Text"=w320) -> ()  [unwired: 2 in, 2 out]
        n128 = local read "Source sweep points"() -> (w314:i32)
        n129 = case shown="1006, Default" "Power ON/Source output function" {
          tunnel: ["I =" ("string") " Vin = " ("string")] -> w305
          frame 1007 {
            # "DC Current"
          }
          frame 1006, Default {
            # "DC Voltage"
          }
        }
        n130 = local read "Load sweep points"() -> (w312:i32)
        n131 = local read "Source sweep values"() -> (w310:dbl[])
        n132 = Build Array("Source enable/disable", "Load enable/disable") -> (w315:bool[])
        n133 = control-ref of="SourceGraph"() -> (w308:refnum<vi>)
        n134 = control-ref of="LoadGraph"() -> (w307:refnum<vi>)
        n135 = Boolean Array To Number(Boolean array=w315) -> (number=w306:u32)
        n136 = case shown="3, Default" w306 {
          tunnel: w314 -> [w358 _ w362]
          tunnel: [1 ("Source sweep points") 1 ("Source sweep points") w362] -> w313
          tunnel: w312 -> [_ w359 w361]
          tunnel: [w358 w359 w361] -> w311
          frame 1 {
            # "Source enabled"
          }
          frame 2 {
            # "Load enabled"
          }
          frame 3, Default {
            # "Both enabled"
          }
        }
        n137 = Build Array(w308, w307) -> (w309:refnum<vi>[])
        n138 = case shown="0, Default" w306 {
          tunnel: w309 -> [w336 w345]
          tunnel: w310 -> [_ w344]
          tunnel: w305 -> [_ w343]
          frame 0, Default {
            n139 = for {
              tunnel: w336 -> [w338] mode=indexing
              n140 = for {
                tunnel: w338 -> [w340]
                tunnel: string[] ["Plot 0", "Plot 1", "Plot 2", "Plot 3", "Plot 4", "Plot 5", "Plot 6", "Plot 7", "Plot 8", "Plot 9", "Plot 10", "Plot 11", "Plot 12", "Plot 13", "Plot 14", "Plot 15", "Plot 16"] -> [w339] mode=indexing
                i -> [w341]
                n141 = To Unsigned Long Integer(number=w341) -> (unsigned 32bit integer=w342:u32)
                n142 = property on="Property Node" class="XYGraph (strict)"(reference=w340, "Active Plot"=w342, "Plot.Plot Name"=w339) -> ()  [unwired: 1 in, 2 out]
              }
            }
          }
          frame 3 {
            # "Both enabled"
            n143 = for {
              tunnel: w345 -> [w348] mode=indexing
              tunnel: w344 -> [w347]
              tunnel: w343 -> [w346]
              n144 = for {
                tunnel: w347 -> [w354] mode=indexing
                tunnel: w348 -> [w351]
                tunnel: w346 -> [w349]
                i -> [w352]
                n145 = Format Value(format string="%.3f", value (0)=w354) -> (output string=w356:string)  [unwired: 1 out]
                n146 = Concatenate Strings(w349, w356) -> (w350:string)
                n147 = To Unsigned Long Integer(number=w352) -> (unsigned 32bit integer=w353:u32)
                n148 = property on="Property Node" class="XYGraph (strict)"(reference=w351, "Active Plot"=w353, "Plot.Plot Name"=w350) -> ()  [unwired: 1 in, 2 out]
              }
            }
          }
        }
        n149 = for {
          N: w313 -> [_]
          tunnel: [w394] -> w331 mode=indexing
          shift-right: [w393] -> _
          shift-left: w328 -> [w390]
          shift-right: [w388] -> _
          shift-left: w326 -> [w389]
          tunnel: w311 -> [w383]
          shift-right: [w381] -> _
          shift-left: w325 -> [w385]
          shift-right: [w380] -> _
          shift-left: w322 -> [w384]
          tunnel: [w379] -> w332 mode=indexing
          w382 = 0 ("index")
          n150 = Delete From Array(array=w390, length=w383, index=w382) -> (deleted portion=w392:dbl[], array with subset deleted=w393:dbl[])
          n151 = Delete From Array(array=w389, length=w383, index=w382) -> (deleted portion=w391:dbl[], array with subset deleted=w388:dbl[])
          n152 = Delete From Array(array=w385, length=w383, index=w382) -> (deleted portion=w386:dbl[], array with subset deleted=w381:dbl[])
          n153 = Delete From Array(array=w384, length=w383, index=w382) -> (deleted portion=w387:dbl[], array with subset deleted=w380:dbl[])
          n154 = Bundle("Source currents"=w392, "Source voltages"=w391) -> (w394:T6)  [unwired: 1 in]
          n155 = Bundle("Load voltages"=w386, "Load currents"=w387) -> (w379:T7)  [unwired: 1 in]
        }
        "LoadGraph" <- w332
        "SourceGraph" <- w331
      }
      frame "Exit" {
        # "This case is triggered to close the User Interface from framework"
        n156 = Flush Queue(queue=w399, error in (no error)=w401) -> (queue out=w398:refnum<queue>, error out=w397:errorcluster)  [unwired: 1 out]
        n157 = Release Queue(queue=w398, force destroy? (F)=TRUE, error in (no error)=w397) -> (error out=w396:errorcluster)  [unwired: 2 out]
      }
      frame "Handle Error" {
      }
    }
  }
